vi "calc.vi"() -> ()   [LabVIEW 2016]
panel:
  out "Error":string
  in  "operation":enum16{"+", "-", "x", "/", "sqrt", "^"}(ring)
  in  "number 2":dbl
  out "ans":dbl
  in  "number 1":dbl
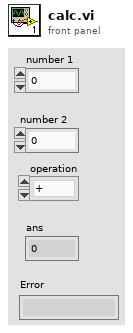
[diagram p1: front panel]
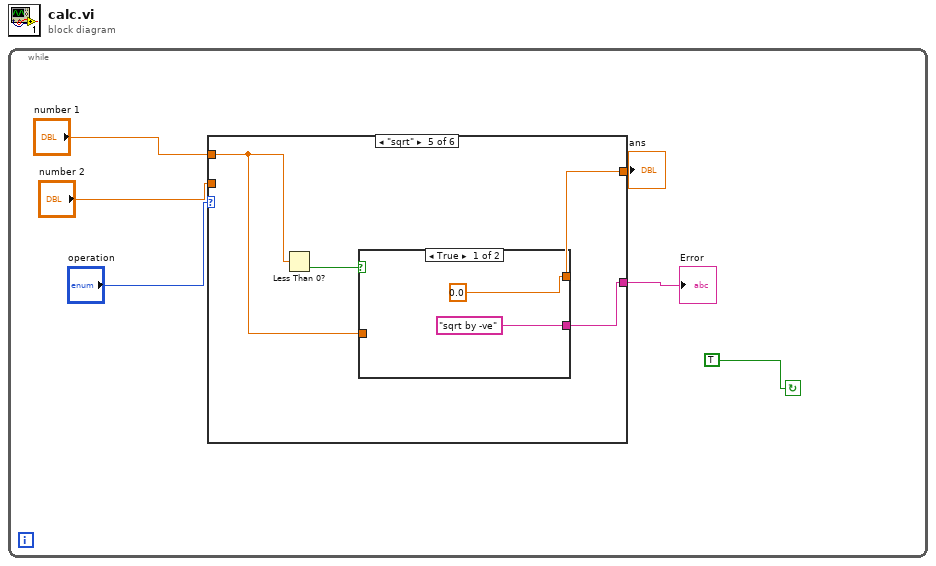
[diagram p0: block diagram]
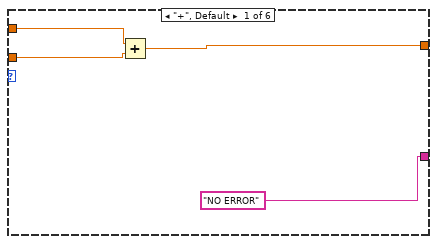
[diagram p2: hidden frame]
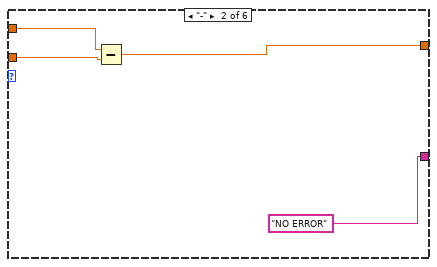
[diagram p3: hidden frame]
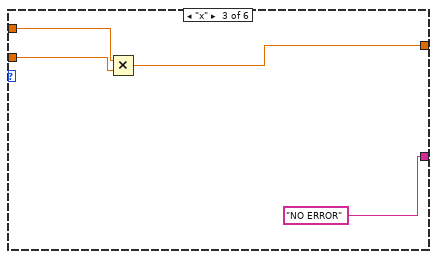
[diagram p4: hidden frame]
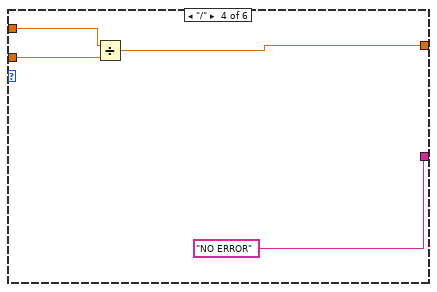
[diagram p5: hidden frame]
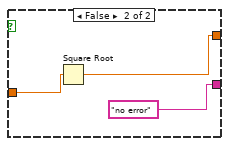
[diagram p6: hidden frame]
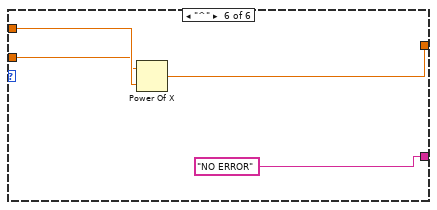
[diagram p7: hidden frame]
diagram:
  n1 = while {
    stop <- TRUE continue-if-true
    n2 = case shown="\"sqrt\"" "operation" {
      tunnel: "number 1" -> [w9 w14 w18 w22 w24 w33]
      tunnel: [w10 w12 w16 w20 w23 w35] -> w5
      tunnel: "number 2" -> [w8 w13 w17 w21 _ w32]
      tunnel: ["NO ERROR" "NO ERROR" "NO ERROR" "NO ERROR" w26 "NO ERROR"] -> w1
      frame "+", Default {
        n3 = Add(x=w9, y=w8) -> (x+y=w10:dbl)
      }
      frame "-" {
        n4 = Subtract(x=w14, y=w13) -> (x-y=w12:dbl)
      }
      frame "x" {
        n5 = Multiply(x=w18, y=w17) -> (x*y=w16:dbl)
      }
      frame "/" {
        n6 = Divide(x=w22, y=w21) -> (x/y=w20:dbl)
      }
      frame "sqrt" {
        n7 = Less Than 0?(x=w24) -> (x < 0?=w25:bool)
        n8 = case shown="True" w25 {
          tunnel: ["sqrt by -ve" "no error"] -> w26
          tunnel: w24 -> [_ w31]
          tunnel: [0.0 w30] -> w23
          frame True {
          }
          frame False {
            n9 = Square Root(x=w31) -> (sqrt(x)=w30:dbl)
          }
        }
      }
      frame "^" {
        n10 = Power Of X(1:w33, 2:w32) -> (0:w35:dbl)
      }
    }
    "ans" <- w5
    "Error" <- w1
  }
